vi "Check LIDAR Ranges.vi"(4 "Magnitude":dbl[](array[numeric])) -> (1 "Magnitude out":dbl[](array[numeric]))   [LabVIEW 2012]
uses:
  Utilities/Robot Parameters/Robot Parameters.vi
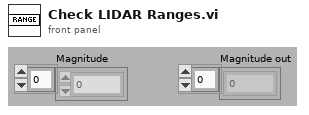
[diagram p1: front panel]
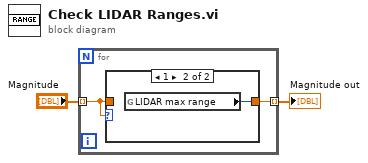
[diagram p0: block diagram]
diagram:
  n1 = for {
    tunnel: "Magnitude" -> [w4] mode=indexing
    tunnel: [w3] -> w1 mode=indexing
    n2 = case shown="1" w4 {
      tunnel: [w5 w6] -> w3
      tunnel: w4 -> [w5 _]
      frame 0, Default {
      }
      frame 1 {
        n3 = global read "Robot Parameters.vi" "LIDAR max range"() -> (w6:i32)
      }
    }
  }
  "Magnitude out" <- w1
